vi "ButtonLanguage.vi"(8 "error in (no error)":errorcluster, 11 "Prooduct Actor in":refnum<class "Prooduct Actor.lvclass">) -> (0 "error out":errorcluster, 3 "Prooduct Actor out":refnum<class "Prooduct Actor.lvclass">)   [LabVIEW 2020, in "Prooduct Actor.lvlib" / "Prooduct Actor.lvclass"]
uses:
  Prooduct Actor.lvclass
  Prooduct Actor.lvclass/Prooduct Actor.ctl
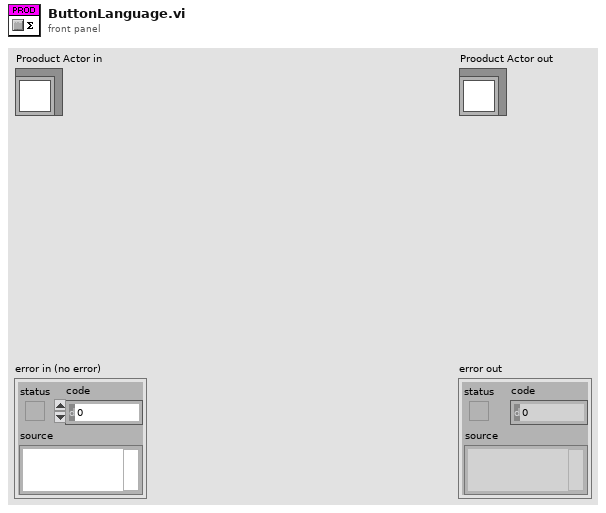
[diagram p1: front panel]
types:
  T1 = typedef "Language Enum.ctl" = enum16{"English", "Español", "Français"}
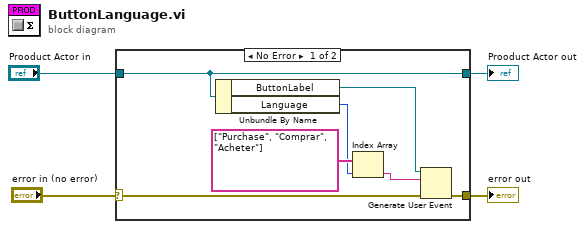
[diagram p0: block diagram]
diagram:
  n1 = case shown="No Error" "error in (no error)" {
    selector: "error in (no error)" -> [w8 w13]
    tunnel: [w7 w13] -> w3
    tunnel: [w10 w12] -> w1
    tunnel: "Prooduct Actor in" -> [w10 w12]
    frame No Error {
      n2 = Unbundle By Name(w10) -> ("ButtonLabel"=w6:refnum<user-event>, "Language"=w9:T1)
      n3 = Index Array(array=string[] ["Purchase", "Comprar", "Acheter"], index=w9) -> (element=w5:string)
      n4 = Generate User Event(user event=w6, event data cluster=w5, error in=w8) -> (error out=w7:errorcluster)  [unwired: 1 in, 1 out]
    }
    frame Error {
    }
  }
  "error out" <- w3
  "Prooduct Actor out" <- w1
